vi "Get Key String.vi"(7 "rel_path":string, 8 "error in (no error)":errorcluster, 9 "default value":string, 10 "key":string, 11 "section":string) -> (0 "error out":errorcluster, 3 "value":string)   [LabVIEW 2016]
uses:
  <vilib>/Utility/config.llb/Read Key (String).vi
  <vilib>/Utility/config.llb/NI_LVConfig.lvlib
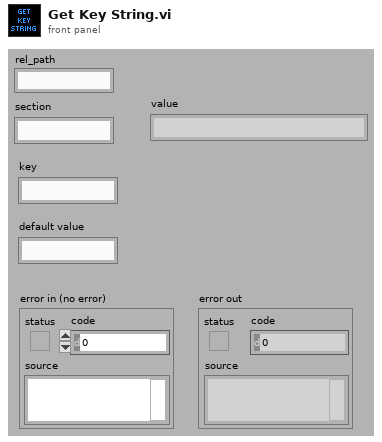
[diagram p1: front panel]
types:
  T1 = enum32{"invalid app kind", "Development System", "Run Time System", "Student Edition", "Embedded LabVIEW", "Evaluation", "Custom"}
  T2 = typedef "NI_LVConfig.lvlib/Config Data RefNum.ctl" = refnum<k1>
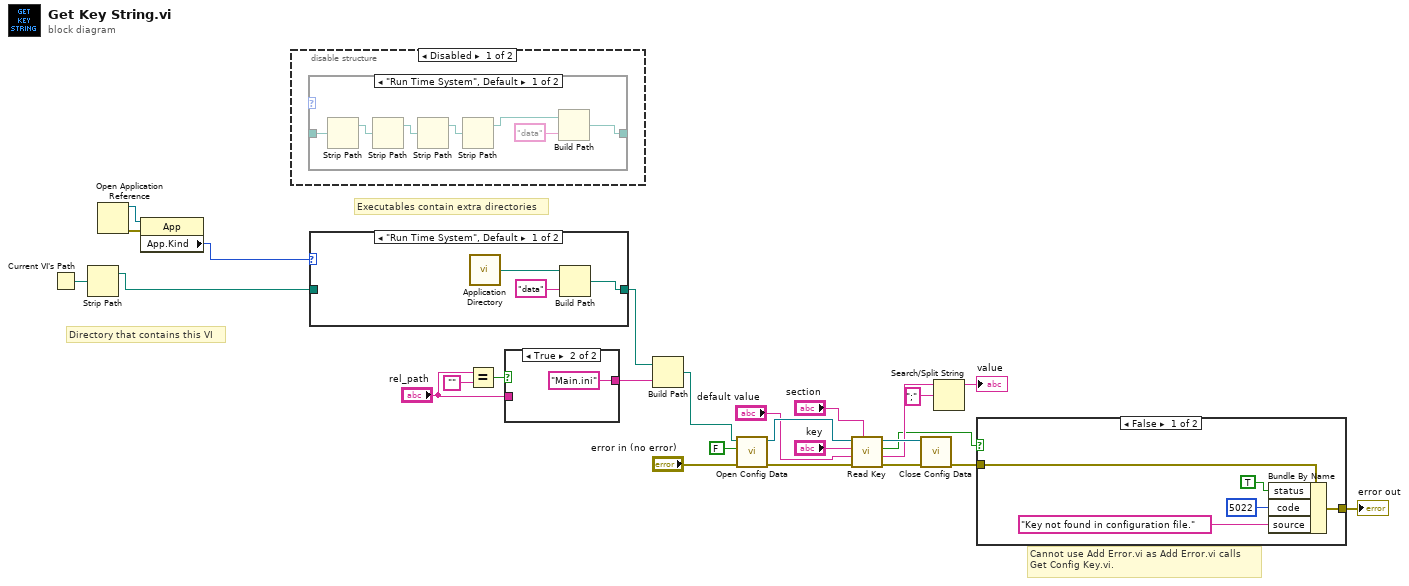
[diagram p0: block diagram]
diagram:
  # "Executables contain extra directories"
  # "Directory that contains this VI"
  # "Cannot use Add Error.vi as Add Error.vi calls\nGet Config Key.vi."
  n1 = Current VI's Path() -> (path=w6:path)
  n2 = Strip Path(path=w6) -> (stripped path=w2:path)  [unwired: 1 out]
  n3 = Open Application Reference() -> (0:w4:errorcluster, 3:w5:refnum<vi>)  [unwired: 4 in]
  n4 = property class="App"(reference=w5, error in=w4) -> ("App.Kind"=w3:T1)  [unwired: 2 out]
  n5 = disable-structure shown="Disabled" {
    frame Disabled {
      n6 = case shown="\"Run Time System\", Default" {
        selector: _ -> [_ _]
        tunnel: _ -> [w27 w34]
        tunnel: [w32 w34] -> _
        frame "Run Time System", Default {
          n7 = Strip Path(path=w27) -> (stripped path=w29:path)  [unwired: 1 out]
          n8 = Strip Path(path=w29) -> (stripped path=w28:path)  [unwired: 1 out]
          n9 = Strip Path(path=w28) -> (stripped path=w33:path)  [unwired: 1 out]
          n10 = Strip Path(path=w33) -> (stripped path=w31:path)  [unwired: 1 out]
          n11 = Build Path(base path=w31, name or relative path="data") -> (appended path=w32:path)
        }
        frame "Development System" {
        }
      }
    }
    frame Enabled {
    }
  }
  n12 = case shown="\"Run Time System\", Default" w3 {
    tunnel: w2 -> [_ w38]
    tunnel: [w37 w38] -> w1
    frame "Run Time System", Default {
      n13 = call <vilib>:"Application Directory.vi"() -> ("Application Directory"=w35:path)
      n14 = Build Path(base path=w35, name or relative path="data") -> (appended path=w37:path)
    }
    frame "Development System" {
    }
  }
  n15 = Equal?(x="rel_path", y="") -> (x = y?=w12:bool)
  n16 = case shown="True" w12 {
    tunnel: [w39 "Main.ini" ("name or relative path")] -> w10
    tunnel: "rel_path" -> [w39 _]
    frame False {
    }
    frame True {
    }
  }
  n17 = Build Path(base path=w1, name or relative path=w10) -> (appended path=w26:path)
  n18 = call <vilib>:"Open Config Data.vi"("error in (no error)"="error in (no error)", "create file if necessary (T)"=FALSE, "configuration file path"=w26) -> ("error out"=w21:errorcluster, "refnum"=w24:T2)  [unwired: 6 in, 1 out]
  n19 = call-poly <vilib>:"Read Key.vi"("section"="section", "error in (no error)"=w21, "default value"="default value", "key"="key", "refnum"=w24) -> ("error out"=w20:errorcluster, "value"=w14:string, "found?"=w7:bool, "refnum out"=w19:T2)  [unwired: 3 in]
  n20 = call <vilib>:"Close Config Data.vi"("error in (no error)"=w20, "refnum"=w19) -> ("error out"=w8:errorcluster)  [unwired: 8 in, 1 out]
  n21 = Search/Split String(string=w14, search string/char (-)=";") -> (substring before match=→"value":string)  [unwired: 1 in, 2 out]
  n22 = case shown="False" w7 {
    tunnel: [w43 w46] -> w9
    tunnel: w8 -> [w41 w46]
    frame False {
      n23 = Bundle By Name(cluster=w41, "status"=TRUE, "code"=5022, "source"="Key not found in configuration file.") -> (w43:errorcluster)
    }
    frame True {
    }
  }
  "error out" <- w9
